vi "DefPnlAndCursor.vi"(7 "AllowDefPan? (T)":bool=TRUE, 8 "error in (no error)":errorcluster, 10 "DeferPanUpdts?":bool, 11 "Tbl Ctrl Refnum":refnum<vi>) -> (0 "error out":errorcluster)   [LabVIEW 2013]
doc: "DeferPanUpdts can greatly speed up front-panel drawing changes. This subVI takes a Table Control reference (Tbl Ctrl Refnum) and optionally (if AllowDefPan?) sets or clears DeferPanUpdts?\nAdditionally, the cursor is changed to \"working\" when updates are deferred.\nYou must set DeferPanUpdts to false again, otherwise the panel will be unresponsive."
uses:
  <vilib>/Utility/cursorutil.llb/Set Cursor (Icon Pict).vi
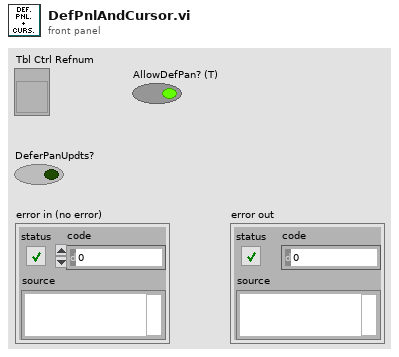
[diagram p1: front panel]
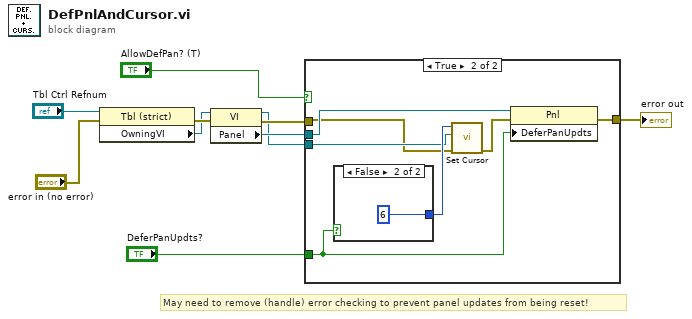
[diagram p0: block diagram]
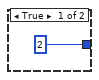
[diagram p3: hidden frame]
diagram:
  # "May need to remove (handle) error checking to prevent panel updates from being reset!"
  n1 = property class="Tbl (strict)"(reference="Tbl Ctrl Refnum", error in="error in (no error)") -> (error out=w7:errorcluster, "OwningVI"=w6:refnum<vi>)  [unwired: 1 out]
  n2 = property class="VI"(reference=w6, error in=w7) -> (reference out=w2:refnum<vi>, error out=w4:errorcluster, "Panel"=w3:refnum<vi>)
  n3 = case shown="True" "AllowDefPan? (T)" {
    tunnel: [w11 w18] -> w10
    tunnel: "DeferPanUpdts?" -> [_ w15]
    tunnel: w4 -> [w11 w12]
    tunnel: w3 -> [_ w14]
    tunnel: w2 -> [_ w13]
    frame False {
    }
    frame True {
      n4 = case shown="False" w15 {
        tunnel: [u16 2 ("icon") u16 6 ("icon")] -> w16
        frame True {
        }
        frame False {
        }
      }
      n5 = call-poly <vilib>:"Set Cursor.vi"("error in (no error)"=w12, "VI reference (current VI)"=w13, "icon"=w16) -> ("error out"=w17:errorcluster)  [unwired: 7 in, 1 out]
      n6 = property class="Pnl"(reference=w14, error in=w17, "DeferPanUpdts"=w15) -> (error out=w18:errorcluster)  [unwired: 1 out]
    }
  }
  "error out" <- w10
